vi "I2C_ReadWrite.vi"(5 "error in (no error)":errorcluster, 7 "DataWriteArray":u8[](array[numeric]) format="%.0x", 8 "Address":u8 max=127 format="%.0x", 9 "Command":enum16{"Write", "Read"}(ring), 11 "RIO Device":T1="RIO0") -> (4 "error out":errorcluster, 6 "Read Data":u8 format="%.0x", 10 "RIO Device out":T1)   [LabVIEW 2018]
uses:
  <vilib>/userdefined/High Color/nirio_resource_hc.ctl
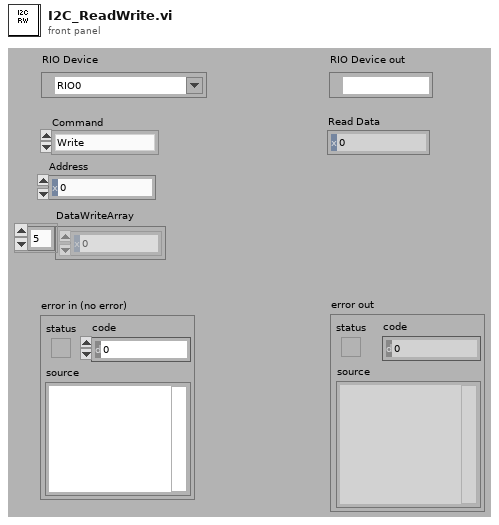
[diagram p1: front panel]
types:
  T1 = typedef "nirio_resource_hc.ctl" = tag
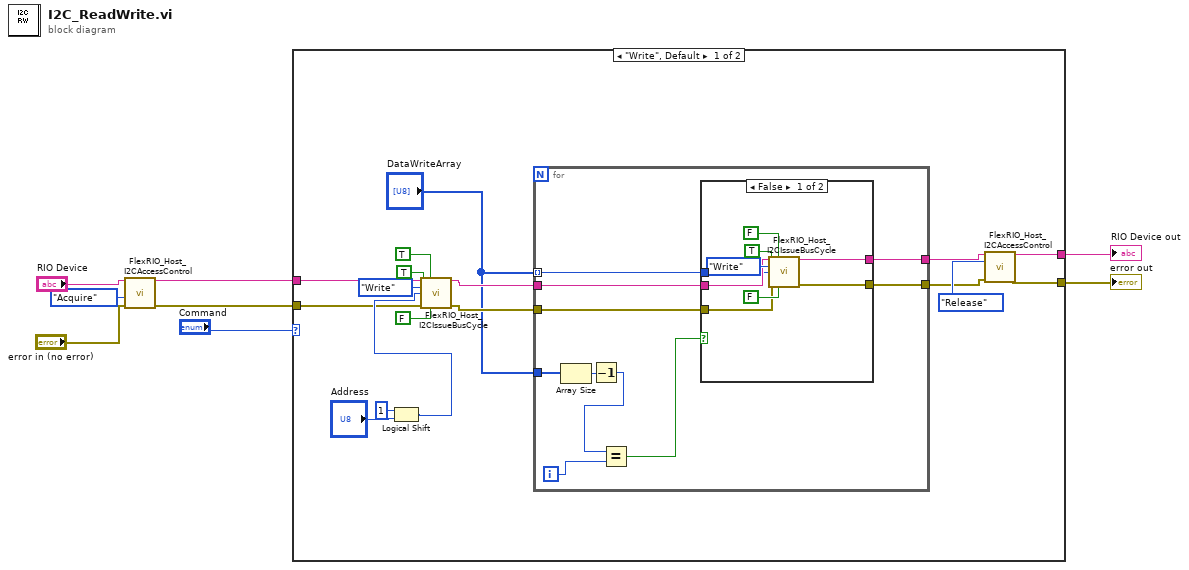
[diagram p0: block diagram]
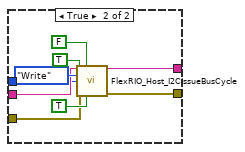
[diagram p2: hidden frame]
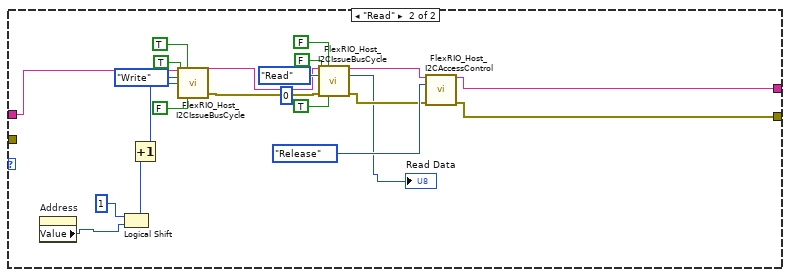
[diagram p3: hidden frame]
diagram:
  n1 = call <vilib>:"FlexRIO_Host_I2CAccessControl.vi"("RIO Device"="RIO Device", "Method"=enum16{"Acquire", "Release"}."Acquire", "error in (no error)"="error in (no error)") -> ("RIO Device out"=w4:T1, "error out"=w1:errorcluster)  [unwired: 11 in]
  n2 = case shown="\"Write\", Default" "Command" {
    tunnel: w4 -> [w25 w71]
    tunnel: [w14 w64] -> w3
    tunnel: [w13 w63] -> w2
    tunnel: w1 -> [w9 _]
    frame "Write", Default {
      n3 = Logical Shift(y=i8 1, x="Address") -> (x << y=w10:u8)
      n4 = call <vilib>:"FlexRIO_Host_I2CIssueBusCycle.vi"("RIO Device"=w25, "Start bit?"=TRUE, "Command"=enum16{"Write", "Read"}."Write", "Write Data"=w10, "Expect Ack?"=TRUE, "error in (no error)"=w9, "Stop bit?"=FALSE) -> ("RIO Device out"=w20:T1, "error out"=w19:errorcluster)  [unwired: 6 in, 1 out]
      n5 = for {
        tunnel: "DataWriteArray" -> [w34] mode=indexing
        tunnel: w20 -> [w35]
        tunnel: w19 -> [w33]
        tunnel: "DataWriteArray" -> [w32]
        tunnel: [w27] -> w17
        tunnel: [w26] -> w15
        i -> [w31]
        n6 = Array Size(array=w32) -> (size(s)=w30:i32)
        n7 = Decrement(x=w30) -> (x-1=w29:i32)
        n8 = Equal?(x=w29, y=w31) -> (x = y?=w28:bool)
        n9 = case shown="False" w28 {
          tunnel: w35 -> [w41 w50]
          tunnel: w34 -> [w40 w49]
          tunnel: w33 -> [w38 w47]
          tunnel: [w37 w46] -> w27
          tunnel: [w36 w45] -> w26
          frame False {
            n10 = call <vilib>:"FlexRIO_Host_I2CIssueBusCycle.vi"("RIO Device"=w41, "Start bit?"=FALSE, "Command"=enum16{"Write", "Read"}."Write", "Write Data"=w40, "Expect Ack?"=TRUE, "error in (no error)"=w38, "Stop bit?"=FALSE) -> ("RIO Device out"=w37:T1, "error out"=w36:errorcluster)  [unwired: 6 in, 1 out]
          }
          frame True {
            n11 = call <vilib>:"FlexRIO_Host_I2CIssueBusCycle.vi"("RIO Device"=w50, "Start bit?"=FALSE, "Command"=enum16{"Write", "Read"}."Write", "Write Data"=w49, "Expect Ack?"=TRUE, "error in (no error)"=w47, "Stop bit?"=TRUE) -> ("RIO Device out"=w46:T1, "error out"=w45:errorcluster)  [unwired: 6 in, 1 out]
          }
        }
      }
      n12 = call <vilib>:"FlexRIO_Host_I2CAccessControl.vi"("RIO Device"=w17, "Method"=enum16{"Acquire", "Release"}."Release", "error in (no error)"=w15) -> ("RIO Device out"=w14:T1, "error out"=w13:errorcluster)  [unwired: 11 in]
    }
    frame "Read" {
      n13 = property on="Address" class="DigNum (strict)"() -> ("Value"=w56:u8)  [unwired: 2 in, 2 out]
      n14 = Logical Shift(y=i8 1, x=w56) -> (x << y=w55:u8)
      n15 = Increment(x=w55) -> (x+1=w54:u8)
      n16 = call <vilib>:"FlexRIO_Host_I2CIssueBusCycle.vi"("RIO Device"=w71, "Start bit?"=TRUE, "Command"=enum16{"Write", "Read"}."Write", "Write Data"=w54, "Expect Ack?"=TRUE, "Stop bit?"=FALSE) -> ("RIO Device out"=w66:T1, "error out"=w65:errorcluster)  [unwired: 7 in, 1 out]
      n17 = call <vilib>:"FlexRIO_Host_I2CIssueBusCycle.vi"("RIO Device"=w66, "Start bit?"=FALSE, "Command"=enum16{"Write", "Read"}."Read", "Write Data"=u8 0, "Expect Ack?"=FALSE, "error in (no error)"=w65, "Stop bit?"=TRUE) -> ("RIO Device out"=w62:T1, "Read Data"=→"Read Data":u8, "error out"=w60:errorcluster)  [unwired: 6 in]
      n18 = call <vilib>:"FlexRIO_Host_I2CAccessControl.vi"("RIO Device"=w62, "Method"=enum16{"Acquire", "Release"}."Release", "error in (no error)"=w60) -> ("RIO Device out"=w64:T1, "error out"=w63:errorcluster)  [unwired: 11 in]
    }
  }
  "RIO Device out" <- w3
  "error out" <- w2
